vi "Git_ProgressFGV.vi"(4 "Action":T1=enum."Update", 6 "Update":u8, 8 "Error In":errorcluster, 9 "Slide in":refnum<vi>) -> (0 "Error Out":errorcluster)   [LabVIEW 2012]
uses:
  Git_ProgressFGV_enum.ctl
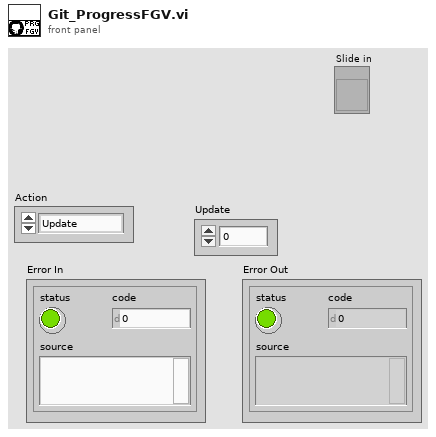
[diagram p1: front panel]
types:
  T1 = typedef "Git_ProgressFGV_enum.ctl" = enum16{"Init", "Update"}
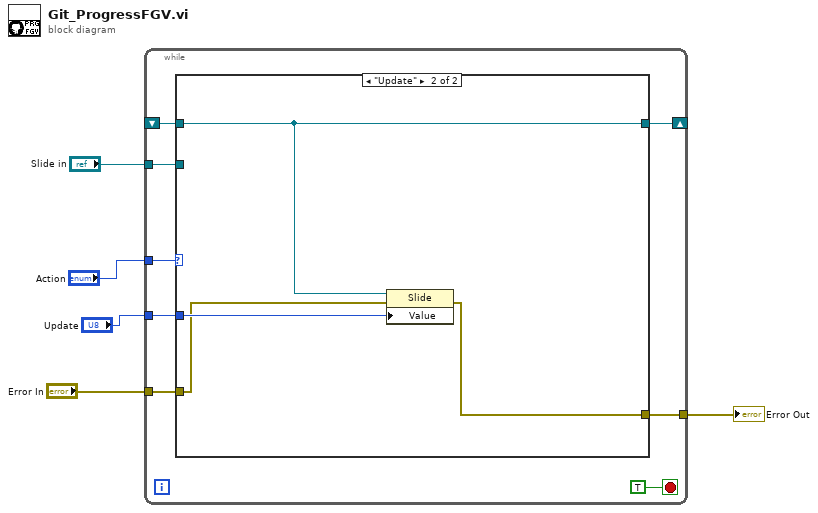
[diagram p0: block diagram]
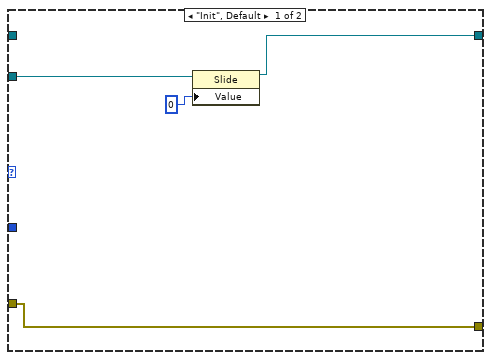
[diagram p2: hidden frame]
diagram:
  n1 = while {
    tunnel: "Slide in" -> [w13]
    shift-right: [w12] -> _
    shift-left: _ -> [w11]
    tunnel: "Action" -> [w10]
    tunnel: "Update" -> [w9]
    tunnel: "Error In" -> [w8]
    tunnel: [w7] -> w1
    stop <- TRUE stop-if-true
    n2 = case shown="\"Update\"" w10 {
      tunnel: w13 -> [w16 _]
      tunnel: [w15 w18] -> w12
      tunnel: w11 -> [_ w18]
      tunnel: w9 -> [_ w21]
      tunnel: w8 -> [w14 w20]
      tunnel: [w14 w19] -> w7
      frame "Init", Default {
        n3 = property class="Slide"(reference=w16, "Value"=u8 0 ("Front Panel Window:Transparency")) -> (reference out=w15:refnum<vi>)  [unwired: 1 in, 1 out]
      }
      frame "Update" {
        n4 = property class="Slide"(reference=w18, error in=w20, "Value"=w21) -> (error out=w19:errorcluster)  [unwired: 1 out]
      }
    }
  }
  "Error Out" <- w1
